vi "DSF.Engine.Transfer Group.Return FIFO.Destroy.vi"(8 "error in (no error)":errorcluster, 11 "Transfer Group in":refnum<class "DSF.Engine.Transfer Group.lvclass">) -> (0 "error out":errorcluster, 3 "Transfer Group out":refnum<class "DSF.Engine.Transfer Group.lvclass">)   [LabVIEW 2017, in "DSF.Engine.lvlib" / "DSF.Engine.Transfer Group.lvclass"]
uses:
  DSF.Engine.Transfer Group.lvclass
  DSF.Engine.Transfer Group.lvclass/DSF.Engine.Transfer Group.ctl
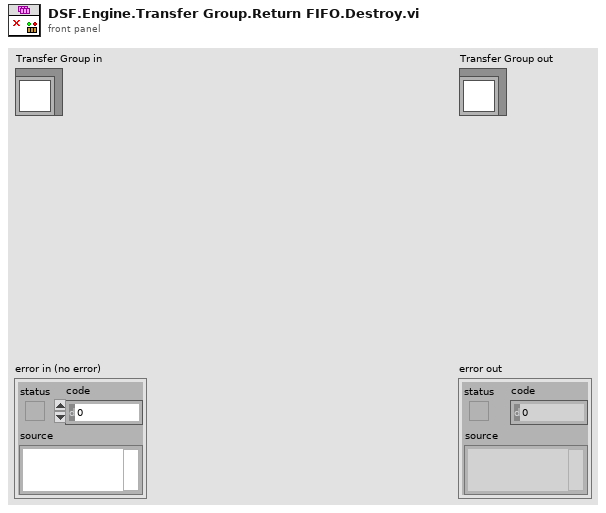
[diagram p1: front panel]
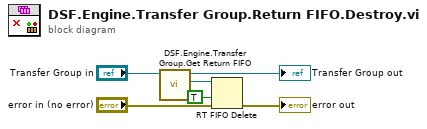
[diagram p0: block diagram]
diagram:
  n1 = call "DSF.Engine.Transfer Group.Get Return FIFO.vi"("Transfer Group in"="Transfer Group in") -> ("Return FIFO"=w3:refnum<k33>, "Transfer Group out"=→"Transfer Group out":refnum<class "DSF.Engine.Transfer Group.lvclass">)  [unwired: 9 in]
  n2 = RT FIFO Delete(0:w3, 2:TRUE ("force destroy? (F)"), 3:"error in (no error)") -> (11:→"error out":errorcluster)
